vi "STM_Server.vi"() -> ()   [LabVIEW 2020, in "RemoteControl.STM.lvclass"]
uses:
  RemoteControl.STM.lvclass
  <vilib>/NI/STM/SubVIs/MetaDataElement.ctl
  <vilib>/NI/STM/TCP/Write Meta Data (TCP Ref).vi
  <vilib>/NI/STM/TCP/Get Connection Reference (TCP).vi
  <vilib>/NI/STM/TCP/Write Meta Data (TCP Clst).vi
  <vilib>/NI/STM/TCP/Read Message (TCP).vi
  <vilib>/NI/STM/TCP/Write Message (TCP).vi
  <vilib>/NI/STM/NI STM.lvlib
panel:
  in  "service name":string
  out "remote address":string
  out "command received":T1
  in  "Enum":T2(ring)
  out "data received":string
  in  "stop":bool
  out "error out":errorcluster
  # "SERVER  (INSTRUMENT)"
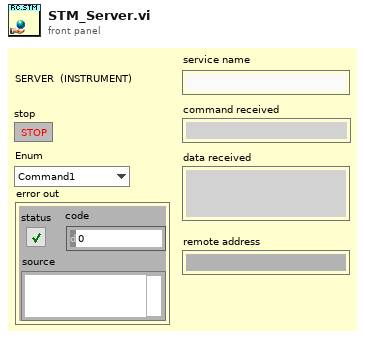
[diagram p1: front panel]
types:
  T1 = typedef "NI STM.lvlib/MetaDataElement.ctl" = string
  T2 = enum16{"Command1", "Command2", "Command3", "Command4", "HELP", "ACK", "CLOSE"}
  T3 = typedef "NI STM.lvlib/TCP Connection Info.ctl" = cluster{"connection ID":refnum<k5>, "meta data":T1[]}
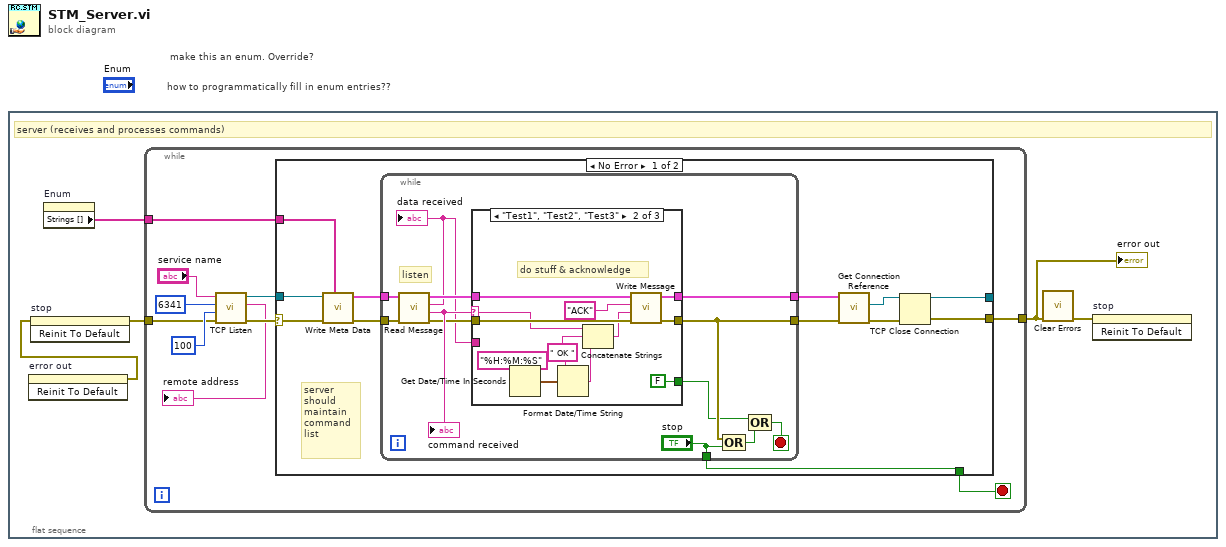
[diagram p0: block diagram]
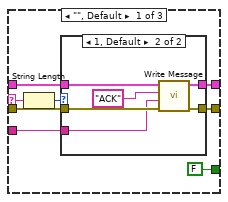
[diagram p2: hidden frame]
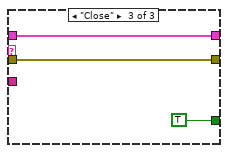
[diagram p4: hidden frame]
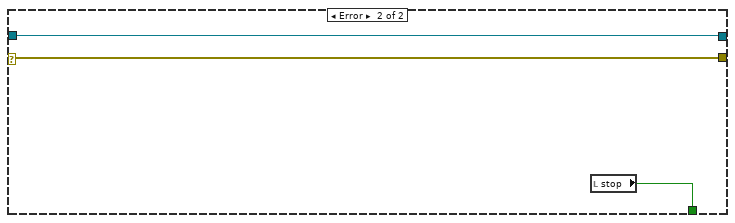
[diagram p5: hidden frame]
diagram:
  # "how to programmatically fill in enum entries??"
  # "make this an enum. Override?"
  n1 = flat-sequence {
    frame #0 {
      # "server (receives and processes commands)"
      n2 = invoke on="error out" class="Clust (strict)" method="Reinit To Default"() -> (error out=w1:errorcluster)  [unwired: 3 in, 2 out]
      n3 = invoke on="stop" class="Bool (strict)" method="Reinit To Default"(error in=w1) -> (error out=w5:errorcluster)  [unwired: 2 in, 2 out]
      n4 = property on="Enum" class="Enum (strict)"() -> ("Strings []"=w2:string[])  [unwired: 2 in, 2 out]
      n5 = while {
        tunnel: w5 -> [w10]
        tunnel: [w9] -> w3
        tunnel: w2 -> [w8]
        stop <- w13 stop-if-true
        n6 = call <vilib>:"TCP Listen.vi"("error in (no error)"=w10, "timeout ms (wait forever: -1)"=100, "port"=u16 6341 ("remote port or service name"), "service name"="service name") -> ("error out"=w11:errorcluster, "remote address"=→"remote address":string, "connection ID"=w14:refnum<k5>)  [unwired: 3 in, 2 out]
        n7 = case shown="No Error" w11 {
          selector: w11 -> [w21 w72]
          tunnel: w14 -> [w20 w71]
          tunnel: [w23 w73] -> w13
          tunnel: [w22 w72] -> w9
          tunnel: w8 -> [w17 _]
          tunnel: [w16 w71] -> _
          frame No Error {
            # "server\nshould \nmaintain\ncommand\nlist"
            n8 = call-poly <vilib>:"Write Meta Data.vi"("meta data"=w17, "error in"=w21, "connection ID"=w20) -> ("error out"=w18:errorcluster, "connection info out"=w19:T3)  [unwired: 7 in]
            n9 = while {
              tunnel: w19 -> [w39]
              tunnel: w18 -> [w38]
              tunnel: [w33] -> w27
              tunnel: [w34] -> w26
              tunnel: ["stop"] -> w23
              stop <- w31 stop-if-true
              # "listen"
              n10 = call-poly <vilib>:"Read Message.vi"("error in"=w38, "connection info in"=w39) -> ("error out"=w36:errorcluster, "name"=w37:T1, "data string"=w28:string, "connection info out"=w35:T3)  [unwired: 4 in, 2 out]
              "data received" <- w28
              "command received" <- w37
              n11 = case shown="\"Test1\", \"Test2\", \"Test3\"" w37 {
                selector: w37 -> [w42 w61 _]
                tunnel: w36 -> [w44 w67 w70]
                tunnel: w35 -> [w46 w66 w69]
                tunnel: [w43 w64 w70] -> w33
                tunnel: [w45 w65 w69] -> w34
                tunnel: [FALSE ("value") FALSE ("value") TRUE ("value")] -> w30
                tunnel: w28 -> [w40 _ _]
                frame "", Default {
                  n12 = String Length(string=w42) -> (length=w41:i32)
                  n13 = case shown="1, Default" w41 {
                    tunnel: w46 -> [w48 w54]
                    tunnel: [w48 w53] -> w45
                    tunnel: w44 -> [w49 w52]
                    tunnel: [w49 w51] -> w43
                    tunnel: w40 -> [_ w50]
                    frame 0 {
                    }
                    frame 1, Default {
                      n14 = call-poly <vilib>:"Write Message.vi"("error in"=w52, "data"=w50, "name"="ACK", "connection info in"=w54) -> ("error out"=w51:errorcluster, "connection info out"=w53:T3)  [unwired: 6 in]
                    }
                  }
                }
                frame "Test1", "Test2", "Test3" {
                  # "do stuff & acknowledge"
                  n15 = Get Date/Time In Seconds() -> (seconds since 1Jan1904=w58:timestamp)
                  n16 = Format Date/Time String(time format string (%c)="%H:%M:%S", seconds (now)=w58) -> (date/time string=w57:string)  [unwired: 1 in]
                  n17 = Concatenate Strings(w61, " OK " ("data"), w57) -> (w60:string)
                  n18 = call-poly <vilib>:"Write Message.vi"("error in"=w67, "data"=w60, "name"="ACK", "connection info in"=w66) -> ("error out"=w64:errorcluster, "connection info out"=w65:T3)  [unwired: 6 in]
                }
                frame "Close" {
                }
              }
              n19 = Compound Arithmetic op=OR(w33, "stop") -> (w32:bool)
              n20 = Compound Arithmetic op=OR(w30, w32) -> (w31:bool)
            }
            n21 = call-poly <vilib>:"Get Connection Reference.vi"("error in"=w27, "connection info in"=w26) -> ("error out"=w25:errorcluster, "connection ID out"=w24:refnum<k5>)  [unwired: 7 in, 1 out]
            n22 = TCP Close Connection(connection ID=w24, error in (no error)=w25) -> (connection ID out=w16:refnum<k5>, error out=w22:errorcluster)  [unwired: 1 in]
          }
          frame Error {
            n23 = local read "stop"() -> (w73:bool)
          }
        }
      }
      "error out" <- w3
      n24 = call <vilib>:"Clear Errors.vi"("error in (no error)"=w3) -> ("error out"=w4:errorcluster)  [unwired: 5 in, 1 out]
      n25 = invoke on="stop" class="Bool (strict)" method="Reinit To Default"(error in=w4) -> ()  [unwired: 2 in, 3 out]
    }
  }
